vi "Flex Readers Demo.vi"() -> ()   [LabVIEW 2020]
uses:
  Flex/Flex.lvlib
panel:
  out "Timed Out?":bool
  out "Slow i":i32
  out "Fast i":i32
  out "Lossy Fast Timeout":bool
  out "Timeout":bool
  in  "Publish Timeout":i32
  in  "Stop 4":bool
  in  "Stop 3":bool
  in  "Stop 2":bool
  in  "Stop 1":bool
  in  "Stop":bool
  out "Lossless Timeout":dbl(graph)
  out "Lossless":dbl(graph)
  out "Lossy Slow/Wait":dbl(graph)
  out "Lossy Fast":dbl(graph)
  in  "Publish Period mS":u32=5
  in  "Slide":dbl(slide)=5.0 scale=0.0..10.0
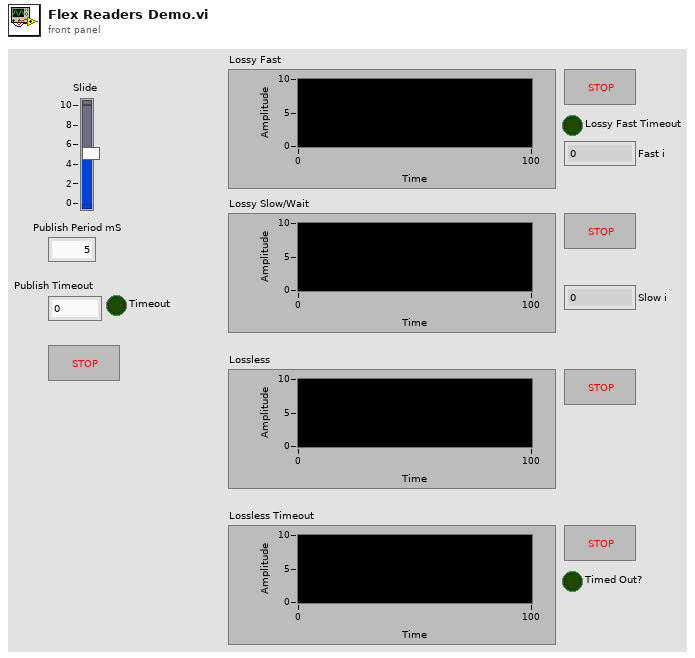
[diagram p1: front panel]
types:
  T1 = typedef "Flex.lvlib/))Channel.ctl" = refnum<queue>
  T2 = typedef "Flex.lvlib/Element.ctl" = dbl
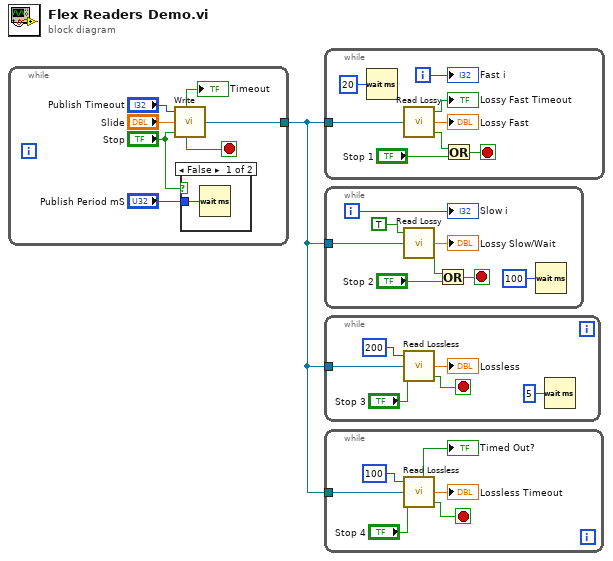
[diagram p0: block diagram]
diagram:
  n1 = while {
    tunnel: [w3] -> w1
    stop <- w4 stop-if-true
    n2 = call "Write.vi"("Timeout mS (-1)"="Publish Timeout", "element"="Slide", "Close? (F)"="Stop") -> ("Timed Out?"=→"Timeout":bool, "Closed?"=w4:bool, "channel"=w3:T1)  [unwired: 2 in]
    n3 = case shown="False" "Stop" {
      tunnel: "Publish Period mS" -> [w9 _]
      frame False {
        n4 = Wait (ms)(milliseconds to wait=w9) -> ()  [unwired: 1 out]
      }
      frame True {
      }
    }
  }
  n5 = while {
    tunnel: w1 -> [w17]
    i -> [w13]
    stop <- w14 stop-if-true
    n6 = Wait (ms)(milliseconds to wait=u32 20) -> ()  [unwired: 1 out]
    n7 = call "Read Lossy.vi"("FlexChannel"=w17) -> ("Timed Out?"=→"Lossy Fast Timeout":bool, "Value"=→"Lossy Fast":T2, "Closed?"=w10:bool)  [unwired: 4 in, 2 out]
    n8 = Or(x=w10, y="Stop 1") -> (x .or. y?=w14:bool)
    "Fast i" <- w13
  }
  n9 = while {
    tunnel: w1 -> [w24]
    i -> [w20]
    stop <- w22 stop-if-true
    n10 = call "Read Lossy.vi"("Wait for Next? (F)"=TRUE, "FlexChannel"=w24) -> ("Value"=→"Lossy Slow/Wait":T2, "Closed?"=w18:bool)  [unwired: 3 in, 3 out]
    n11 = Or(x=w18, y="Stop 2") -> (x .or. y?=w22:bool)
    n12 = Wait (ms)(milliseconds to wait=u32 100) -> ()  [unwired: 1 out]
    "Slow i" <- w20
  }
  n13 = while {
    tunnel: w1 -> [w31]
    stop <- w28 stop-if-true
    n14 = call "Read Lossless.vi"("Depth (Unlimited)"=200, "FlexChannel"=w31, "Release (F)"="Stop 3") -> ("Element"=→"Lossless":T2, "Closed?"=w28:bool)  [unwired: 4 in, 1 out]
    n15 = Wait (ms)(milliseconds to wait=u32 5) -> ()  [unwired: 1 out]
  }
  n16 = while {
    tunnel: w1 -> [w34]
    stop <- w33 stop-if-true
    n17 = call "Read Lossless.vi"("Timeout mS (-1)"=100, "FlexChannel"=w34, "Release (F)"="Stop 4") -> ("Timed Out?"=→"Timed Out?":bool, "Element"=→"Lossless Timeout":T2, "Closed?"=w33:bool)  [unwired: 4 in]
  }
